vi "MP-285 Set Origin.vi"(2 "error in (no error)":errorcluster, 3 "VISA resource name":refnum<visa-resource-name>) -> (0 "error out":errorcluster, 1 "VISA resource name out":refnum<visa-resource-name>)   [LabVIEW 2010]
uses:
  StageMG100204SutterMP285/StageMG100204SutterMP285.lvclass
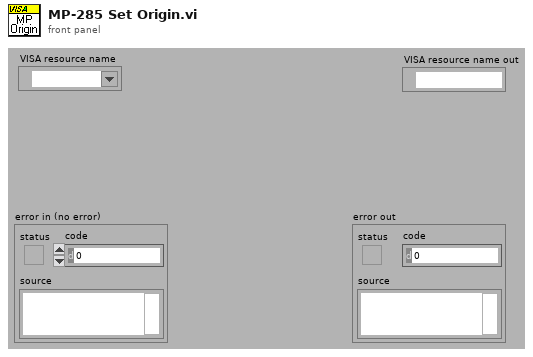
[diagram p1: front panel]
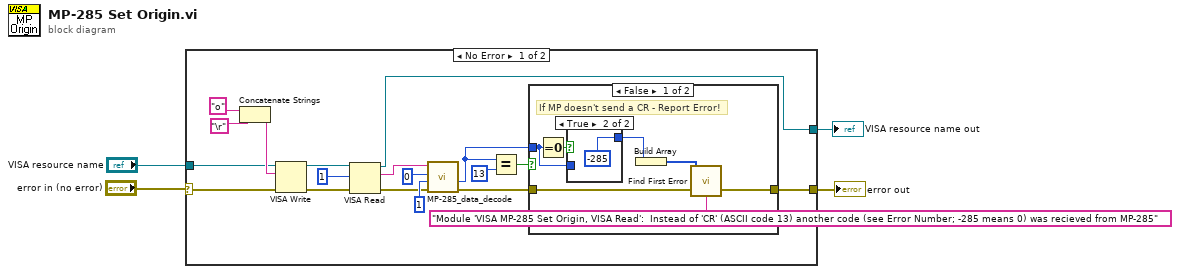
[diagram p0: block diagram]
diagram:
  n1 = case shown="No Error" "error in (no error)" {
    selector: "error in (no error)" -> [w9 w34]
    tunnel: [w12 w33] -> w4
    tunnel: [w11 w34] -> w3
    tunnel: "VISA resource name" -> [w10 w33]
    frame No Error {
      n2 = Concatenate Strings("o", "\r") -> (w20:string)
      n3 = VISA Write(VISA resource name=w10, write buffer=w20, error in (no error)=w9) -> (VISA resource name out=w19:refnum<visa-resource-name>, error out=w18:errorcluster)  [unwired: 1 out]
      n4 = VISA Read(VISA resource name=w19, byte count=u32 1, error in (no error)=w18) -> (VISA resource name out=w12:refnum<visa-resource-name>, read buffer=w13:string, error out=w6:errorcluster)  [unwired: 1 out]
      n5 = call "MP-285_data_decode.vi"("error in (no error)"=w6, "length"=1, "offset"=0, "encoded data string in"=w13) -> ("error out"=w5:errorcluster, "decoded data"=w7:i32)  [unwired: 5 in, 1 out]
      n6 = Equal?(x=w7, y=13) -> (x = y?=w15:bool)
      n7 = case shown="False" w15 {
        tunnel: [w29 w32] -> w11
        tunnel: w7 -> [w25 _]
        tunnel: w5 -> [w23 w32]
        frame False {
          # "If MP doesn't send a CR - Report Error!"
          n8 = Equal To 0?(x=w25) -> (x = 0?=w26:bool)
          n9 = case shown="True" w26 {
            tunnel: w25 -> [w30 _]
            tunnel: [w30 -285] -> w24
            frame False {
            }
            frame True {
            }
          }
          n10 = Build Array(w24) -> (w27:i32[])
          n11 = call <vilib>:"Find First Error.vi"("error in (no error)"=w23, "source messages"="Module 'VISA MP-285 Set Origin, VISA Read':  Instead of 'CR' (ASCII code 13) another code (see Error Number; -285 means 0) was recieved from MP-285", "error codes"=w27) -> ("error out"=w29:errorcluster)  [unwired: 2 out]
        }
        frame True {
          # "TRUE: CR was received - NO Errors"
        }
      }
    }
    frame Error {
    }
  }
  "VISA resource name out" <- w4
  "error out" <- w3
